vi "T12.vi"(2 "Parametry Ziemi":T1={"a - półoś duża"=6378137.0, "b - półoś mała"=6356752.3141999999998} {"b - półoś mała" format="%_20f"; "a - półoś duża" format="%_20g"}, 3 "fi'":ext) -> (7 "T12":ext)   [LabVIEW 2015, in "Biblioteka moduł map v3.lvlib" / "Konwersja wsp.lvlib" / "UTM.lvlib" / "Konwersja z UTM na wsp geograficzne.lvlib"]
uses:
  Konwersja z UTM na wsp geograficzne.lvlib
  UTM.lvlib
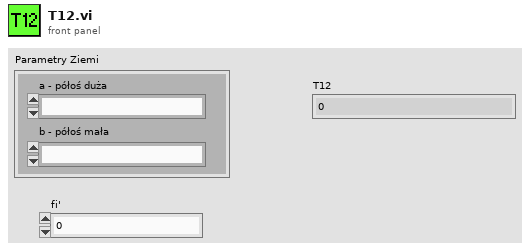
[diagram p1: front panel]
types:
  T1 = cluster{"a - półoś duża":ext, "b - półoś mała":ext}
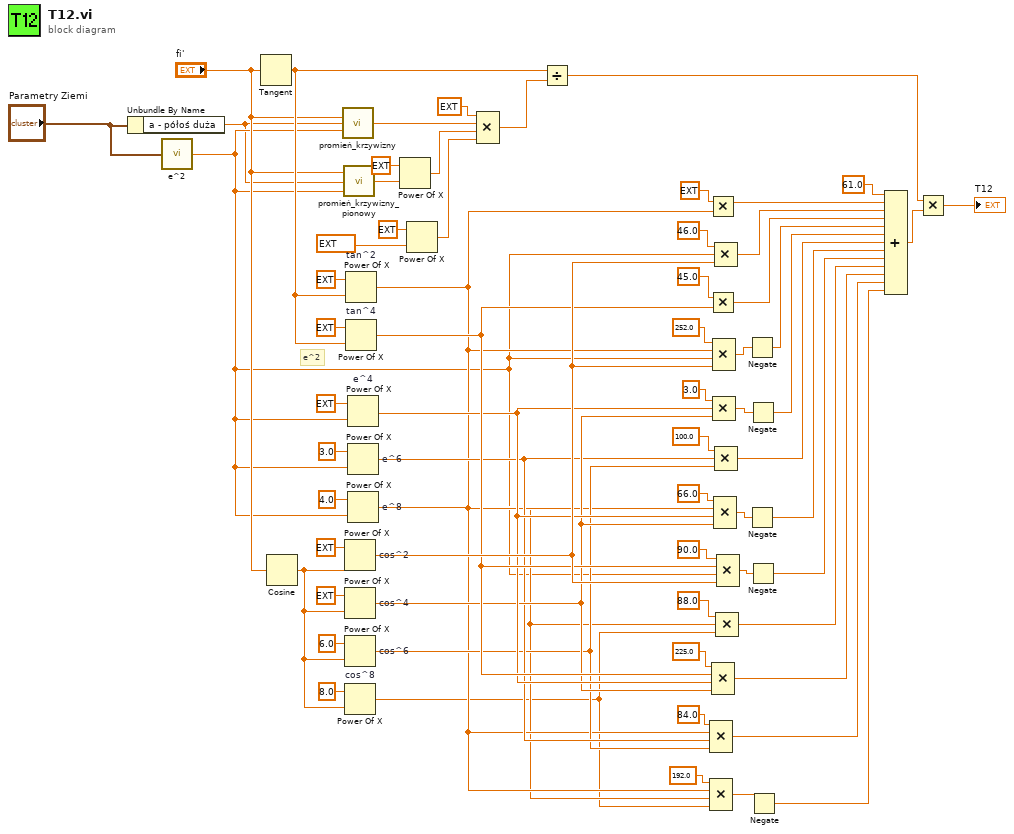
[diagram p0: block diagram]
diagram:
  # "e^2"
  n1 = Unbundle By Name("Parametry Ziemi") -> ("a - półoś duża"=w1:ext)
  n2 = call "e^2.vi"("Parametry Ziemi"="Parametry Ziemi") -> ("e^2"=w3:ext)  [unwired: 4 in]
  n3 = Tangent(1:"fi'") -> (0:w54:ext)
  n4 = Cosine(x="fi'") -> (cos(x)=w43:ext)
  n5 = call "promień_krzywizny.vi"("e^2"=w3, "a"=w1, "fi[rad]"="fi'") -> ("Promien krzywizny południka"=w64:ext)  [unwired: 2 in]
  n6 = call "promień_krzywizny_pionowy.vi"("e^2"=w3, "a"=w1, "fi[rad]"="fi'") -> ("Promien krzywizny równoleżnika"=w63:dbl)  [unwired: 2 in]
  n7 = Power Of X "cos^2"(1:w43, 2:ext 2.0 ("y")) -> (0:w21:ext)
  n8 = Power Of X "cos^4"(1:w43, 2:ext 4.0 ("y")) -> (0:w14:ext)
  n9 = Power Of X "cos^6"(1:w43, 2:6.0 ("y")) -> (0:w10:ext)
  n10 = Power Of X "cos^8"(1:w43, 2:8.0 ("y")) -> (0:w4:ext)
  n11 = Power Of X "tan^2"(1:w54, 2:ext 2.0 ("y")) -> (0:w6:ext)
  n12 = Power Of X "tan^4"(1:w54, 2:ext 4.0 ("y")) -> (0:w16:ext)
  n13 = Power Of X "e^4"(1:w3, 2:ext 2.0 ("y")) -> (0:w15:ext)
  n14 = Power Of X "e^6"(1:w3, 2:3.0 ("y")) -> (0:w11:ext)
  n15 = Power Of X "e^8"(1:w3, 2:4.0 ("y")) -> (0:w5:ext)
  n16 = Power Of X(1:w63, 2:ext 5.0 ("y")) -> (0:w59:ext)
  n17 = Power Of X(1:ext 0.9996 ("k0"), 2:ext 6.0 ("y")) -> (0:w58:ext)
  n18 = Compound Arithmetic op=MULTIPLY(ext 720.0 ("value"), w64, w59, w58) -> (w66:ext)
  n19 = Divide(x=w54, y=w66) -> (x/y=w57:ext)
  n20 = Multiply(x=ext 90.0, y=w6) -> (x*y=w40:ext)
  n21 = Multiply(x=45.0, y=w16) -> (x*y=w36:ext)
  n22 = Compound Arithmetic op=MULTIPLY(84.0 ("value"), w6, w11, w10) -> (w12:ext)
  n23 = Compound Arithmetic op=MULTIPLY(192.0 ("value"), w6, w5, w4) -> (w9:ext)
  n24 = Compound Arithmetic op=MULTIPLY(225.0 ("value"), w16, w15, w14) -> (w17:ext)
  n25 = Compound Arithmetic op=MULTIPLY(252.0 ("value"), w6, w3, w21) -> (w34:ext)
  n26 = Compound Arithmetic op=MULTIPLY(3.0 ("value"), w15, w14) -> (w31:ext)
  n27 = Compound Arithmetic op=MULTIPLY(66.0 ("value"), w6, w15, w14) -> (w23:ext)
  n28 = Compound Arithmetic op=MULTIPLY(46.0 ("value"), w3, w21) -> (w38:ext)
  n29 = Compound Arithmetic op=MULTIPLY(100.0 ("value"), w11, w10) -> (w28:ext)
  n30 = Compound Arithmetic op=MULTIPLY(88.0 ("value"), w5, w4) -> (w19:ext)
  n31 = Compound Arithmetic op=MULTIPLY(90.0 ("value"), w16, w3, w21) -> (w25:ext)
  n32 = Negate(x=w34) -> (-x=w35:ext)
  n33 = Negate(x=w23) -> (-x=w26:ext)
  n34 = Negate(x=w31) -> (-x=w30:ext)
  n35 = Negate(x=w25) -> (-x=w22:ext)
  n36 = Negate(x=w9) -> (-x=w8:ext)
  n37 = Compound Arithmetic op=ADD(61.0 ("value"), w40, w38, w36, w35, w30, w28, w26, w22, w19, w17, w12, w8) -> (w55:ext)
  n38 = Multiply(x=w57, y=w55) -> (x*y=→"T12":ext)
